vi "Initialize.vi"(8 "error in (no error)":errorcluster, 9 "Reset (True)":bool=TRUE, 10 "ID Query (True)":bool=TRUE, 11 "VISA resource name":refnum<visa-resource-name>) -> (0 "error out":errorcluster, 3 "VISA resource name out":refnum<visa-resource-name>)   [LabVIEW 2023, in "Keysight-DSQx3014T.lvlib"]
doc: "Establishes communication with the instrument and optionally performs an instrument identification query and/or an instrument reset. It also places the instrument in a default state needed for other instrument driver operations. Therefore, call this VI before calling other instrument driver VIs for this instrument. Generally, you need to call the Initialize VI only once at the beginning of an application."
uses:
  Keysight-DSQx3014T.lvlib
  Private/Extended User Data.ctl
  <vilib>/regexp/Match Regular Expression.xnode
panel:
  # "(c) 2011-2017 National Instruments.  ALL RIGHTS RESERVED."
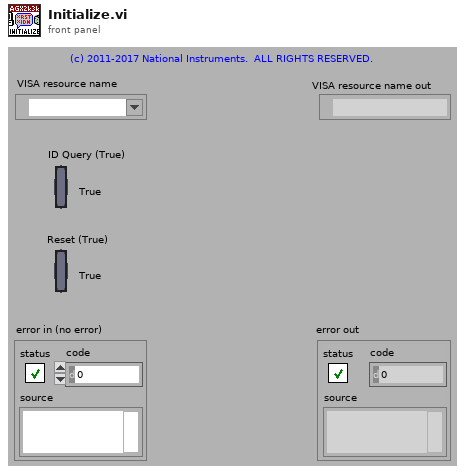
[diagram p1: front panel]
types:
  T1 = typedef "Keysight-DSQx3014T.lvlib/Extended User Data.ctl" = cluster{"X-Series Mode":u16, "Acquisition Type (0: Normal)":i32}
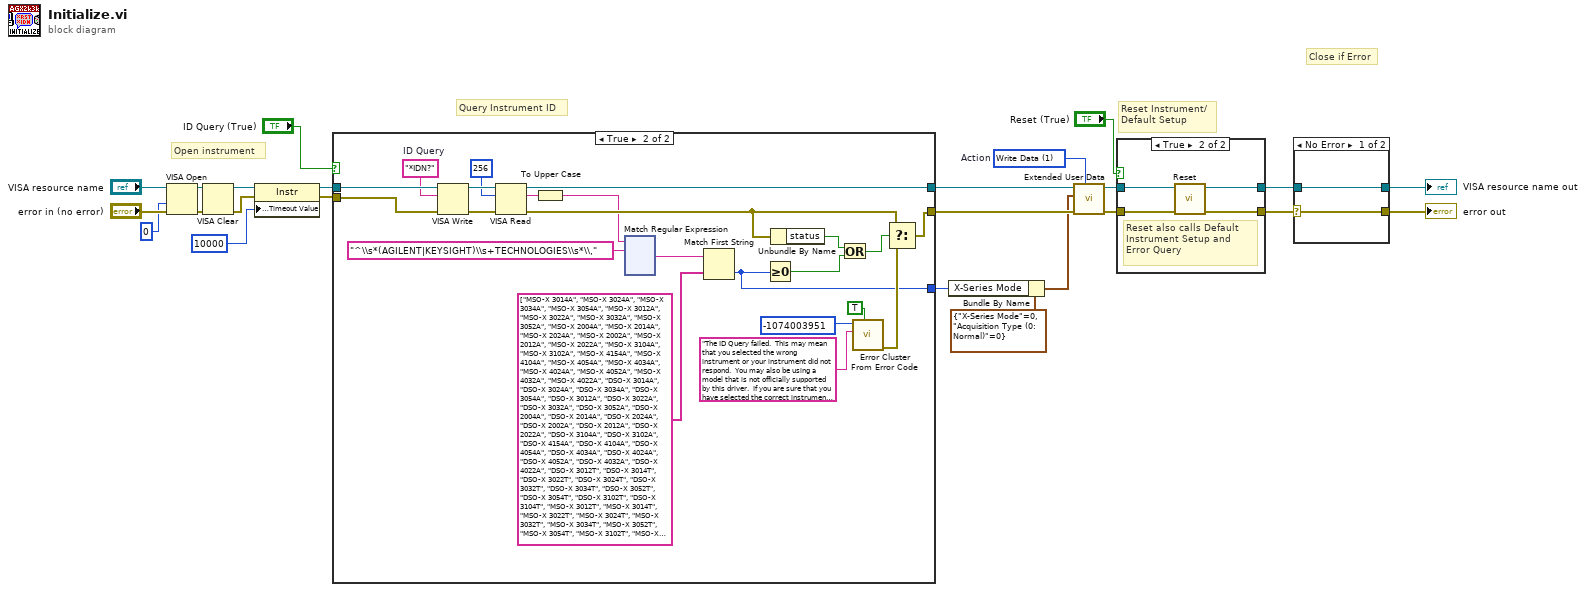
[diagram p0: block diagram]
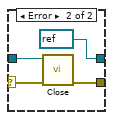
[diagram p2: hidden frame]
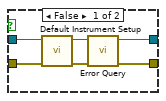
[diagram p3: hidden frame]
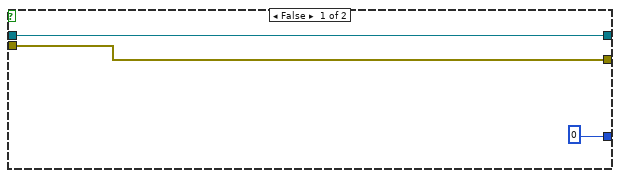
[diagram p4: hidden frame]
diagram:
  w8 = 1 items=["Read Data", "Write Data", "Clear Data", "Clear ALL Data"]  # Action
  # "Close if Error"
  # "Query Instrument ID"
  # "Reset Instrument/\nDefault Setup"
  # "Open instrument"
  n1 = VISA Open(access mode=u32 0, error in (no error)="error in (no error)", VISA resource name="VISA resource name") -> (VISA resource name=w18:refnum<visa-resource-name>, error out=w17:errorcluster)  [unwired: 2 out]
  n2 = VISA Clear(VISA resource name=w18, error in (no error)=w17) -> (VISA resource name out=w16:refnum<visa-resource-name>, error out=w15:errorcluster)
  n3 = property class="Instr"(reference=w16, error in=w15, "General Settings:Timeout Value"=u32 10000) -> (reference out=w10:refnum<visa-resource-name>, error out=w9:errorcluster)
  n4 = case shown="True" "ID Query (True)" {
    tunnel: [w26 w49] -> w5
    tunnel: [w27 w47] -> w7
    tunnel: w10 -> [w27 w48]
    tunnel: w9 -> [w26 w34]
    tunnel: [u16 0 ("X-Series Mode") w33] -> w2
    frame False {
    }
    frame True {
      w43 = "*IDN?"  # ID Query
      n5 = VISA Write(VISA resource name=w48, write buffer=w43, error in (no error)=w34) -> (VISA resource name out=w46:refnum<visa-resource-name>, error out=w45:errorcluster)  [unwired: 1 out]
      n6 = VISA Read(VISA resource name=w46, byte count=u32 256, error in (no error)=w45) -> (VISA resource name out=w47:refnum<visa-resource-name>, read buffer=w32:string, error out=w38:errorcluster)  [unwired: 1 out]
      n7 = To Upper Case(1:w32) -> (0:w29:string)
      n8 = xnode "Match Regular Expression"("input string"=w29, "regular expression"="^\\s*(AGILENT|KEYSIGHT)\\s+TECHNOLOGIES\\s*\\," ("Company Name Regular Expression")) -> ("after match"=w28:string)  [unwired: 4 in, 4 out]
      n9 = Match First String(2:string[] ["MSO-X 3014A", "MSO-X 3024A", "MSO-X 3034A", "MSO-X 3054A", "MSO-X 3012A", "MSO-X 3022A", "MSO-X 3032A", "MSO-X 3052A", "MSO-X 2004A", "MSO-X 2014A", "MSO-X 2024A", "MSO-X 2002A", "MSO-X 2012A", "MSO-X 2022A", "MSO-X 3104A", "MSO-X 3102A", "MSO-X 4154A", "MSO-X 4104A", "MSO-X 4054A", "MSO-X 4034A", "MSO-X 4024A", "MSO-X 4052A", "MSO-X 4032A", "MSO-X 4022A", "DSO-X 3014A", "DSO-X 3024A", "DSO-X 3034A", "DSO-X 3054A", "DSO-X 3012A", "DSO-X 3022A", "DSO-X 3032A", "DSO-X 3052A", "DSO-X 2004A", "DSO-X 2014A", "DSO-X 2024A", "DSO-X 2002A", "DSO-X 2012A", "DSO-X 2022A", "DSO-X 3104A", "DSO-X 3102A", "DSO-X 4154A", "DSO-X 4104A", "DSO-X 4054A", "DSO-X 4034A", "DSO-X 4024A", "DSO-X 4052A", "DSO-X 4032A", "DSO-X 4022A", "DSO-X 3012T", "DSO-X 3014T", "DSO-X 3022T", "DSO-X 3024T", "DSO-X 3032T", "DSO-X 3034T", "DSO-X 3052T", "DSO-X 3054T", "DSO-X 3102T", "DSO-X 3104T", "MSO-X 3012T", "MSO-X 3014T", "MSO-X 3022T", "MSO-X 3024T", "MSO-X 3032T", "MSO-X 3034T", "MSO-X 3052T", "MSO-X 3054T", "MSO-X 3102T", "MSO-X 3104T", "DSO-X 6002A", "DSO-X 6004A", "MSO-X 6002A", "MSO-X 6004A", "EDU-X 1002A", "EDU-X 1002G", "DSO-X 1102A", "DSO-X 1102G"], 3:w28) -> (0:w33:i32)  [unwired: 1 out]
      n10 = Greater Or Equal To 0?(x=w33) -> (x >= 0?=w36:bool)
      n11 = Unbundle By Name(w38) -> ("status"=w37:bool)
      n12 = Or(x=w37, y=w36) -> (x .or. y?=w35:bool)
      n13 = call <vilib>:"Error Cluster From Error Code.vi"("show call chain? (False)"=TRUE, "error message (\"\")"="The ID Query failed.  This may mean that you selected the wrong instrument or your instrument did not respond.  You may also be using a model that is not officially supported by this driver.  If you are sure that you have selected the correct instrument and it is responding, try disabling the ID Query." ("Source (VI Name)"), "error code (0)"=-1074003951 ("Code")) -> ("error out"=w42:errorcluster)  [unwired: 1 in, 5 out]
      n14 = Select(t=w38, s=w35, f=w42) -> (s? t:f=w49:errorcluster)
    }
  }
  n15 = Bundle By Name(cluster=T1 {"X-Series Mode"=0, "Acquisition Type (0: Normal)"=0} ("User Data Definition"), "X-Series Mode"=w2) -> (w3:T1)
  n16 = call "Extended User Data.vi"("Action (1: Write Data)"=w8, "error in (no error)"=w5, "User Data In"=w3, "VISA resource name in"=w7) -> ("error out"=w4:errorcluster, "VISA resource name out"=w6:refnum<visa-resource-name>)  [unwired: 6 out]
  n17 = case shown="True" "Reset (True)" {
    tunnel: w4 -> [w171 w173]
    tunnel: [w168 w176] -> w11
    tunnel: w6 -> [w172 w174]
    tunnel: [w169 w175] -> w12
    frame False {
      n18 = call "Default Instrument Setup.vi"("error in (no error)"=w171, "VISA resource name"=w172) -> ("error out"=w167:errorcluster, "VISA resource name out"=w170:refnum<visa-resource-name>)  [unwired: 8 out]
      n19 = call "Error Query.vi"("error in (no error)"=w167, "VISA resource name"=w170) -> ("error out"=w168:errorcluster, "VISA resource name out"=w169:refnum<visa-resource-name>)  [unwired: 8 out]
    }
    frame True {
      # "Reset also calls Default Instrument Setup and Error Query"
      n20 = call "Reset.vi"("error in (no error)"=w173, "VISA resource name"=w174) -> ("error out"=w176:errorcluster, "VISA resource name out"=w175:refnum<visa-resource-name>)  [unwired: 8 out]
    }
  }
  n21 = case shown="No Error" w11 {
    selector: w11 -> [w177 w180]
    tunnel: w12 -> [w178 w181]
    tunnel: [w178 refnum<visa-resource-name> refnum ("VISA resource name out")] -> w14
    tunnel: [w177 w182] -> w13
    frame No Error {
    }
    frame Error {
      n22 = call "Close.vi"("error in (no error)"=w180, "VISA resource name"=w181) -> ("error out"=w182:errorcluster)  [unwired: 9 out]
    }
  }
  "VISA resource name out" <- w14
  "error out" <- w13
